vi "Write INL Values.vi"(8 "Error in":errorcluster, 10 "INL Values":dbl[](array[numeric]), 11 "INL DNL Test in":refnum<class "INL DNL Test.lvclass">) -> (0 "Error out":errorcluster, 3 "INL DNL Test out":refnum<class "INL DNL Test.lvclass">)   [LabVIEW 2020, in "INL DNL Test.lvclass"]
uses:
  INL DNL Test.lvclass
  INL DNL Test.lvclass/INL DNL Test.ctl
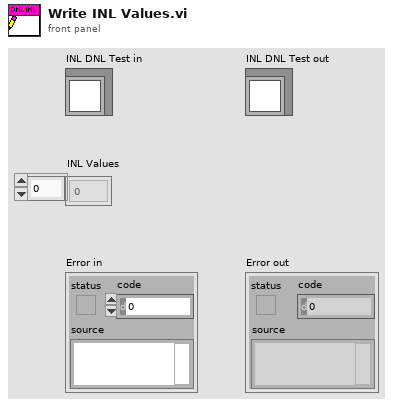
[diagram p1: front panel]
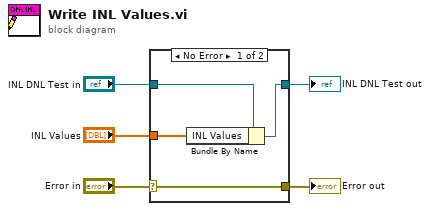
[diagram p0: block diagram]
diagram:
  n1 = case shown="No Error" "Error in" {
    selector: "Error in" -> [w9 w10]
    tunnel: [w9 w10] -> w4
    tunnel: [w7 w11] -> w2
    tunnel: "INL DNL Test in" -> [w8 w11]
    tunnel: "INL Values" -> [w6 _]
    frame No Error {
      n2 = Bundle By Name(cluster=w8, "INL Values"=w6) -> (w7:refnum<class "INL DNL Test.lvclass">)
    }
    frame Error {
    }
  }
  "Error out" <- w4
  "INL DNL Test out" <- w2
